vi "Create Class Icons.vi"(8 "error in (no error)":errorcluster, 11 "QControl Creation in":refnum<class "QControl Creation.lvclass">) -> (0 "error out":errorcluster, 2 "Class Data Icon":refnum<class "Icon.lvclass">, 3 "Class Banner Icon":refnum<class "Icon.lvclass">)   [LabVIEW 2015, in "QControl Creation.lvclass"]
doc: "<b> </b> <b> </b>\n©2016 Q Software Innovations, LLC (QSI)\nwritten by Quentin Alldredge\nproduced in LabVIEW 2015\n\nsupport@qsoftwareinnovations.com\nwww.qsoftwareinnovations.com\n\nAll rights reserved.\n\nRedistribution and use in source and binary forms, with or without modification, are permitted provided that the following conditions are met:\n\n * Redistributions of source code must retain the above copyright notice, this list of conditions and the following disclaimer.\n * Redistributions in binary form must reproduce the above copyright notice, this list of conditions and the following disclaimer in the documentation and/or other materials provided with the distribution.\n * Neither the name of Q Software Innovations, LLC. nor the names of its contributors may be used to endorse or promote products derived from this software without specific prior written permission.\n\nTHIS SOFTWARE IS PROVIDED BY THE COPYRIGHT HOLDERS AND CONTRIBUTORS \"AS IS\" AND ANY EXPRESS OR IMPLIED WARRANTIES, INCLUDING, BUT NOT LIMITED TO, THE IMPLIED WARRANTIES OF MERCHANTABILITY AND FITNESS FOR A PARTICULAR PURPOSE ARE DISCLAIMED. IN NO EVENT SHALL THE COPYRIGHT OWNER OR CONTRIBUTORS BE LIABLE FOR ANY DIRECT, INDIRECT, INCIDENTAL, SPECIAL, EXEMPLARY, OR CONSEQUENTIAL DAMAGES (INCLUDING, BUT NOT LIMITED TO, PROCUREMENT OF SUBSTITUTE GOODS OR SERVICES; LOSS OF USE, DATA, OR PROFITS; OR BUSINESS INTERRUPTION) HOWEVER CAUSED AND ON ANY THEORY OF LIABILITY, WHETHER IN CONTRACT, STRICT LIABILITY, OR TORT (INCLUDING NEGLIGENCE OR OTHERWISE) ARISING IN ANY WAY OUT OF THE USE OF THIS SOFTWARE, EVEN IF ADVISED OF THE POSSIBILITY OF SUCH DAMAGE."
uses:
  QControl Creation.lvclass
  <vilib>/LabVIEW Icon API/lv_icon/Classes/Icon/Icon.lvclass
  <vilib>/LabVIEW Icon API/LabVIEW Icon API.lvlib
  <vilib>/LabVIEW Icon API/API_Rectangle Dimension.ctl
  <vilib>/LabVIEW Icon API/API_Text.ctl
  <vilib>/LabVIEW Icon API/API_Text Colors.ctl
  <vilib>/LabVIEW Icon API/lv_icon/Controls/Alignment.ctl
  <vilib>/LabVIEW Icon API/API_Test Settings.ctl
  <vilib>/picture/picture.llb/imagedata.ctl
  <vilib>/Utility/miscctls.llb/LVPoint32TypeDef.ctl
  <vilib>/LabVIEW Icon API/API_User Layer Data.ctl
  New QControl Info/New QControl Info.lvclass
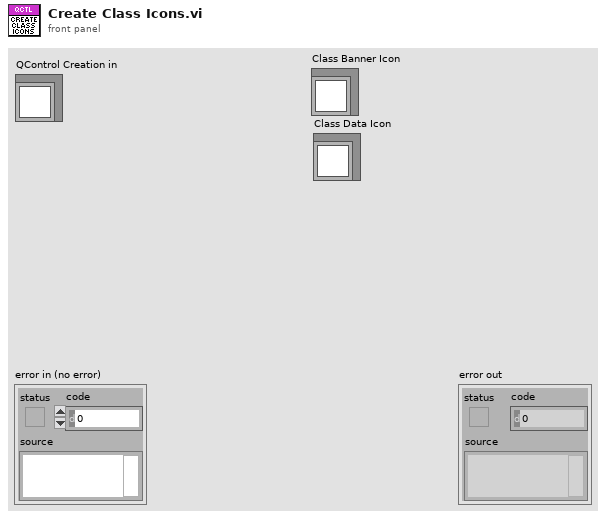
[diagram p1: front panel]
types:
  T1 = typedef "LabVIEW Icon API.lvlib/API_User Layer Data.ctl" = cluster{"Layer name":string, "Origin":T2, "Icon image data":T3}
  T2 = typedef "LVPoint32TypeDef.ctl" = cluster{"Horizontal":i32, "Vertical":i32}
  T3 = typedef "imagedata.ctl" = cluster{"image type":i32, "image depth":i32, "image":u8[], "mask":u8[], "colors":u32[], "Rectangle":cluster{"left":i16, "top":i16, "right":i16, "bottom":i16}}
  T4 = typedef "LabVIEW Icon API.lvlib/API_Test Settings.ctl" = cluster{"Font":string, "Alignment":T5, "Size":u8, "Center text":bool, "Capitalize text":bool, "Text color":T6}
  T5 = typedef "Alignment.ctl" = u16
  T6 = typedef "LabVIEW Icon API.lvlib/API_Text Colors.ctl" = cluster{"Line 1 color":u32, "Line 2 color":u32, "Line 3 color":u32, "Line 4 color":u32}
  T7 = typedef "LabVIEW Icon API.lvlib/API_Text.ctl" = cluster{"Line 1 text":string, "Line 2 text":string, "Line 3 text":string, "Line 4 text":string}
  T8 = typedef "LabVIEW Icon API.lvlib/API_Rectangle Dimension.ctl" = cluster{"Width":i16, "Height":i16}
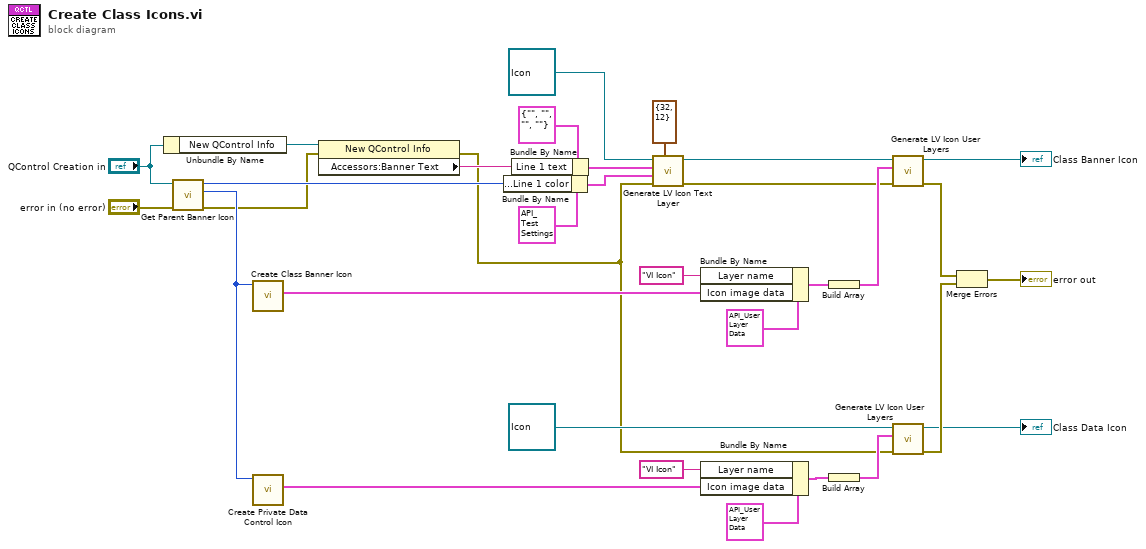
[diagram p0: block diagram]
diagram:
  n1 = Unbundle By Name("QControl Creation in") -> ("New QControl Info"=w32:refnum<data-value>)
  n2 = call "Get Parent Banner Icon.vi"("error in (no error)"="error in (no error)", "QControl Creation in"="QControl Creation in") -> ("error out"=w2:errorcluster, "Banner BG Color"=w5:u32, "Banner Text Color"=w6:u32)  [unwired: 7 in]
  n3 = call "Create Class Banner Icon.vi"("Theme Color"=w5) -> ("Icon Out"=w24:T3)  [unwired: 9 in, 1 out]
  n4 = call "Create Private Data Control Icon.vi"("Theme Color"=w5) -> ("Icon Out"=w17:T3)  [unwired: 9 in, 1 out]
  n5 = property class="New QControl Info"(reference=w32, error in=w2) -> (error out=w1:errorcluster, "Accessors:Banner Text"=w3:string)  [unwired: 1 out]
  n6 = Bundle By Name(cluster=T4 {"Font"="Small Fonts", "Alignment"=1, "Size"=8, "Center text"=TRUE, "Capitalize text"=TRUE, "Text color"={"Line 1 color"=0, "Line 2 color"=0, "Line 3 color"=0, "Line 4 color"=0}} ("Text settings"), "Text color.Line 1 color"=w6) -> (w27:T4)
  n7 = Bundle By Name(cluster=T7 {"Line 1 text"="", "Line 2 text"="", "Line 3 text"="", "Line 4 text"=""} ("Text"), "Line 1 text"=w3) -> (w28:T7)
  n8 = call <vilib>:"Generate LV Icon Text Layer.vi"("Rectangle dimension (32,32)"=T8 {"Width"=32, "Height"=12}, "error in (no error)"=w1, "Text settings"=w27, "Text"=w28, "Icon in"=refnum<class "Icon.lvclass"> refnum ("Icon.lvclass in")) -> ("error out"=w19:errorcluster, "Icon out"=w22:refnum<class "Icon.lvclass">)  [unwired: 5 in]
  n9 = Bundle By Name(cluster=T1 {"Layer name"="", "Origin"={"Horizontal"=0, "Vertical"=0}, "Icon image data"={"image type"=0, "image depth"=0, "image"=[], "mask"=[], "colors"=[], "Rectangle"={"left"=0, "top"=0, "right"=0, "bottom"=0}}} ("User layer"), "Layer name"="VI Icon", "Icon image data"=w24) -> (w21:T1)
  n10 = Bundle By Name(cluster=T1 {"Layer name"="", "Origin"={"Horizontal"=0, "Vertical"=0}, "Icon image data"={"image type"=0, "image depth"=0, "image"=[], "mask"=[], "colors"=[], "Rectangle"={"left"=0, "top"=0, "right"=0, "bottom"=0}}} ("User layer"), "Layer name"="VI Icon", "Icon image data"=w17) -> (w14:T1)
  n11 = Build Array(w21) -> (w20:T1[])
  n12 = Build Array(w14) -> (w15:T1[])
  n13 = call <vilib>:"Generate LV Icon User Layers.vi"("error in (no error)"=w19, "User layers"=w20, "Icon in"=w22) -> ("error out"=w12:errorcluster, "Icon out"=→"Class Banner Icon":refnum<class "Icon.lvclass">)  [unwired: 7 in]
  n14 = call <vilib>:"Generate LV Icon User Layers.vi"("error in (no error)"=w1, "User layers"=w15, "Icon in"=refnum<class "Icon.lvclass"> refnum ("Icon.lvclass in")) -> ("error out"=w11:errorcluster, "Icon out"=→"Class Data Icon":refnum<class "Icon.lvclass">)  [unwired: 7 in]
  n15 = Merge Errors(w12, w11) -> (→"error out":errorcluster)
